vi "HDF5_Init_Tone_Refs_20171218_1427.vi"(5 "HDF5 file ref":T2 format="%.0x", 9 "File Exists?":bool, 11 "error in":errorcluster) -> (3 "ComplexRefs":T1[](array[typedef]) {"Group_ref" format="%.0x"; "QSpect_dset" format="%.0x"; "ISpect_dset" format="%.0x"; "PwrSpect_dset" format="%.0x"; "TImeStamp_dset" format="%.0x"}, 4 "ToneRefs":T3[](array[typedef]) {"Group_ref" format="%.0x"; "Cal"."Downshift_dset" format="%.0x"; "Cal"."DeltaPhase_dset" format="%.0x"; "Cal"."Phase_dset" format="%.0x"; "Cal"."SNR_dset" format="%.0x"; "Cal"."df_dset" format="%.0x"; "Cal"."PeakLoc_dset" format="%.0x"; "Cal"."MaxValue_dset" format="%.0x"; "Cal"."TImeStamp_dset" format="%.0x"; "Cal"."TimeString_dset" format="%.0x"; "Beac"."Downshift_dset" format="%.0x"; "Beac"."DeltaPhase_dset" format="%.0x"; "Beac"."Phase_dset" format="%.0x"; "Beac"."SNR_dset" format="%.0x"; "Beac"."df_dset" format="%.0x"; "Beac"."PeakLoc_dset" format="%.0x"; "Beac"."MaxValue_dset" format="%.0x"; "Beac"."TImeStamp_dset" format="%.0x"; "Beac"."TimeString_dset" format="%.0x"; "CalZoom_dSet" format="%.0x"; "BeacZoom_dSet" format="%.0x"}, 6 "HDF5 file ref":T2 format="%.0x", 15 "error out":errorcluster)   [LabVIEW 2018]
doc: "Set up the HDF5 data structure and initialize the references for the Tone1, Tone2, Tone3, and Tone4 Groups and the datasets (tables) within each Group.\n\nData structure:\nTone1 (Group) \n Beac - cluster (Dataset)\n BeacZoom - 1024 element Double array (waveform) \n Cal - cluster\n CalZoom - 1024 element Double array (waveform) \nTone2\n Beac - cluster\n BeacZoom - 1024 element Double array (waveform) \n Cal - cluster\n CalZoom - 1024 element Double array (waveform) \nTone3\n Beac - cluster\n BeacZoom - 1024 element Double array (waveform) \n Cal - cluster\n CalZoom - 1024 element Double array (waveform) \nTone4\n Beac - cluster\n BeacZoom - 1024 element Double array (waveform) \n Cal - cluster\n CalZoom - 1024 element Double array (waveform)"
uses:
  Controls/Clusts/ToneGroupRefsClust.ctl
  <vilib>/addons/h5labview2/base/hid_t.ctl
  HDF5_Tone_refs.ctl
  HDF5_Complex_Refs.ctl
  lib_path_mod_20200519.vi
  <vilib>/addons/h5labview2/base/H5Equery.vi
  <vilib>/addons/h5labview2/attrib/H5Awrite.llb/H5Awrite.xnode
  <vilib>/addons/h5labview2/group/H5G.lvlib
  <vilib>/addons/h5labview2/dataset/H5D.lvlib
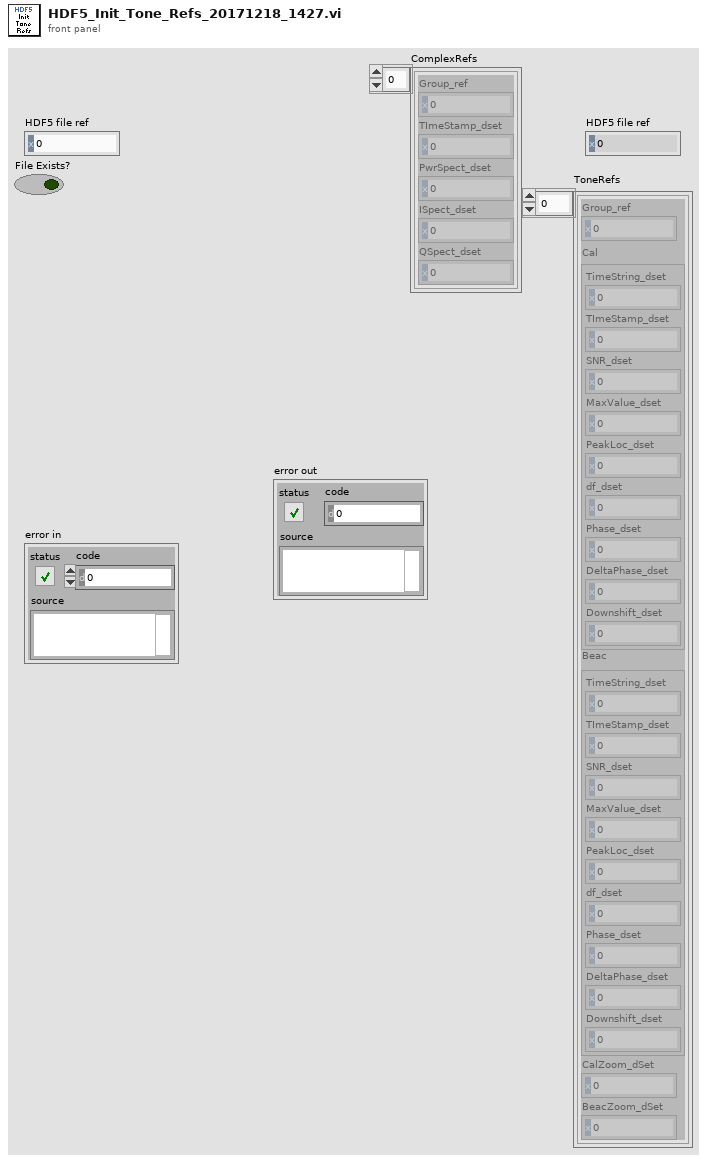
[diagram p1: front panel]
types:
  T1 = typedef "HDF5_Complex_Refs.ctl" = cluster{"Group_ref":T2, "TImeStamp_dset":T2, "PwrSpect_dset":T2, "ISpect_dset":T2, "QSpect_dset":T2}
  T2 = typedef "hid_t.ctl" = i32
  T3 = typedef "ToneGroupRefsClust.ctl" = cluster{"Group_ref":T2, "Cal":T4, "Beac":T4, "CalZoom_dSet":T2, "BeacZoom_dSet":T2}
  T4 = typedef "HDF5_Tone_refs.ctl" = cluster{"TimeString_dset":T2, "TImeStamp_dset":T2, "SNR_dset":T2, "MaxValue_dset":T2, "PeakLoc_dset":T2, "df_dset":T2, "Phase_dset":T2, "DeltaPhase_dset":T2, "Downshift_dset":T2}
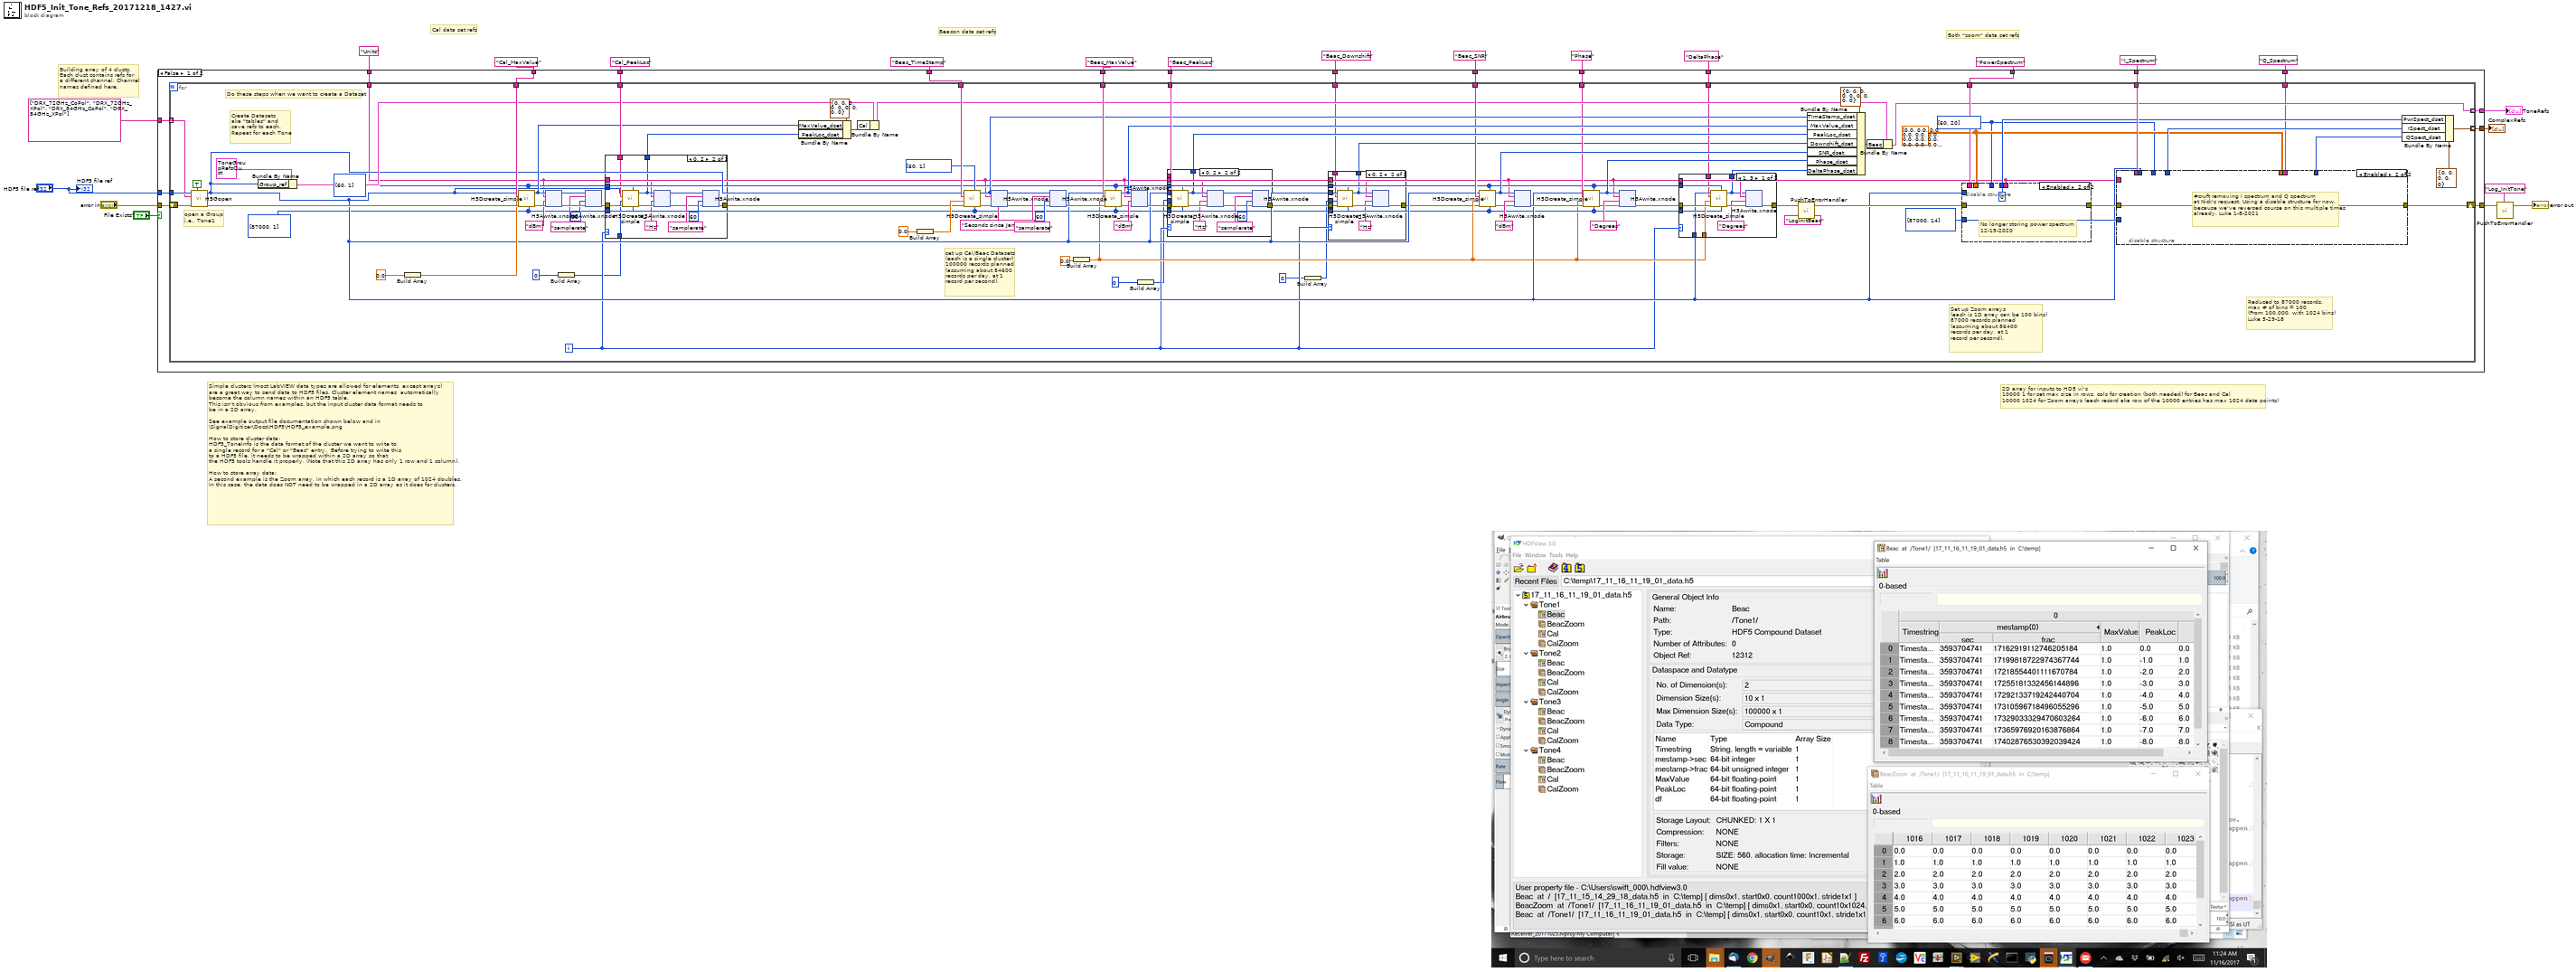
[diagram p0: block diagram]
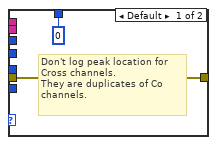
[diagram p2: hidden frame]
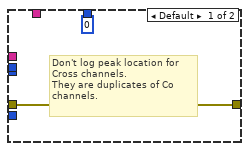
[diagram p3: hidden frame]
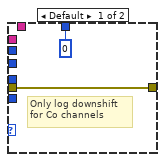
[diagram p4: hidden frame]
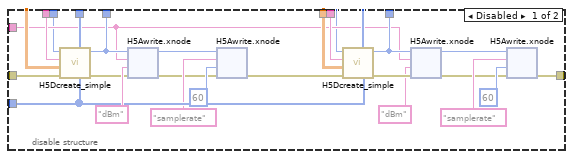
[diagram p5: hidden frame]
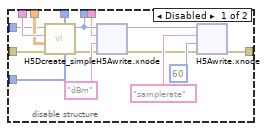
[diagram p6: hidden frame]
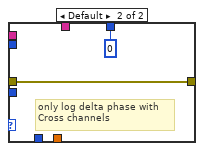
[diagram p7: hidden frame]
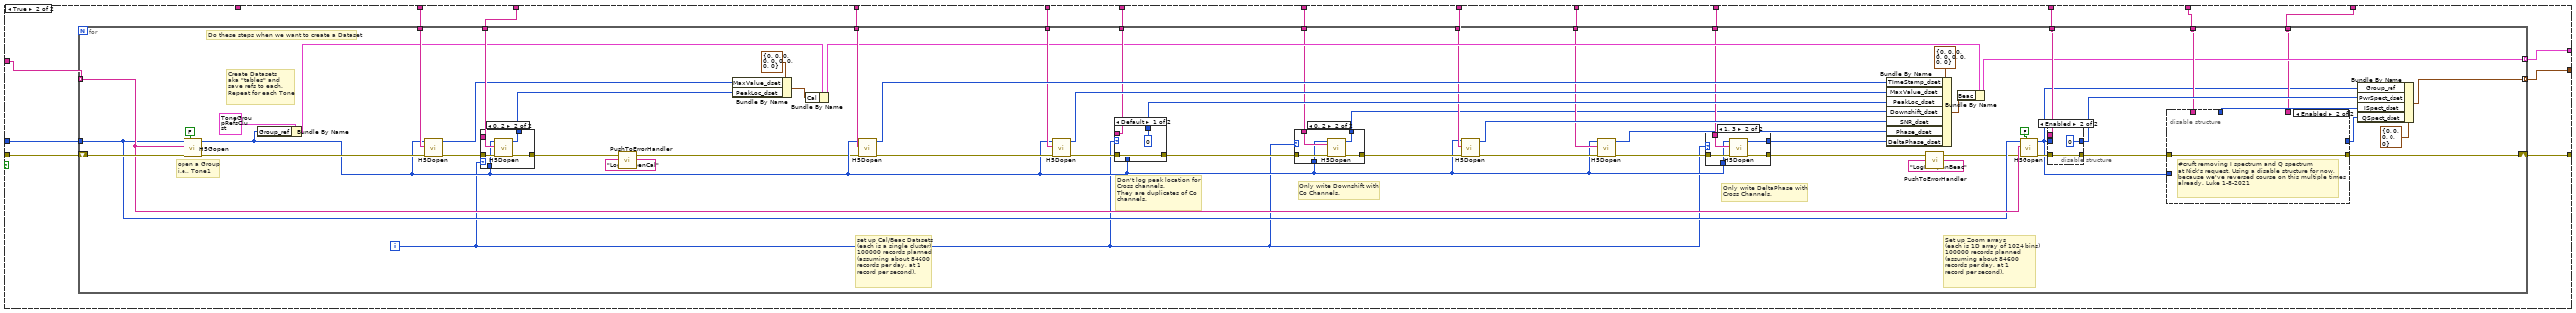
[diagram p8: hidden frame]
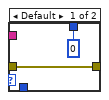
[diagram p9: hidden frame]
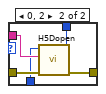
[diagram p10: hidden frame]
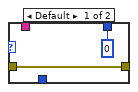
[diagram p11: hidden frame]
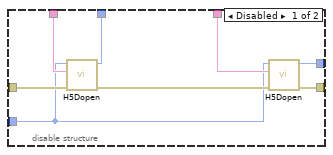
[diagram p12: hidden frame]
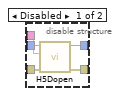
[diagram p13: hidden frame]
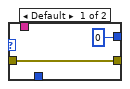
[diagram p14: hidden frame]
diagram:
  # "Both \"zoom\" data set refs"
  # "Beacon data set refs"
  # "Cal data set refs"
  # "Building array of 4 clusts.\nEach clust contains refs for \na different channel. Channel\nnames defined here."
  # "Simple clusters (most LabVIEW data types are allowed for elements, except arrays) \nare a great way to send data to HDF5 files. Cluster element names  automatically\nbecome the column names within an HDF5 table.\nThis isn't obvious from examples, but the input cluster data format needs to \nbe in a 2D array.\n\nSee example output file documentation shown below and in\n\\SignalDigitizer\\Docs\\HDF5\\HDF5_example.png\n\nHow to store cluster data:\nHDF5_ToneInfo is the data format of the cluster we want to write to \na single record for a \"Cal\" or \"Beac\" entry.  Before trying to write this \nto a HDF5 file, it needs to be wrapped within a 2D array so that \nthe HDF5 tools handle it properly. (Note that this 2D array has only 1 row and 1 column).\n\nHow to store array data:\nA second example is the Zoom array, in which each record is a 1D array of 1024 doubles.\nIn this case, the data does NOT need to be wrapped in a 2D array as it does for clusters."
  # "2D array for inputs to HD5 vi's\n10000 1 for set max size in rows, cols for creation (both needed) for Beac and Cal\n10000 1024 for Zoom arrays (each record aka row of the 10000 entries has max 1024 data points)"
  n1 = case shown="False" "File Exists?" {
    tunnel: [w41 w613] -> w22
    tunnel: "error in" -> [w40 w612]
    tunnel: "HDF5 file ref" -> [w39 w611]
    tunnel: string[] ["DRX_72GHz_CoPol", "DRX_72GHz_XPol", "DRX_84GHz_CoPol", "DRX_84GHz_XPol"] -> [w38 w610]
    tunnel: [w37 w609] -> w7
    tunnel: "PowerSpectrum" ("string") -> [w36 w608]
    tunnel: "I_Spectrum" ("string") -> [w35 w607]
    tunnel: "Cal_MaxValue" ("string") -> [w34 w606]
    tunnel: "Cal_PeakLoc" ("string") -> [w33 w605]
    tunnel: "Beac_TimeStamp" ("string") -> [w32 w604]
    tunnel: "Beac_MaxValue" ("string") -> [w31 w603]
    tunnel: "Beac_PeakLoc" ("string") -> [w30 w602]
    tunnel: "Units" ("attrib name") -> [w29 _]
    tunnel: [w28 w601] -> w9
    tunnel: "Q_Spectrum" ("string") -> [w27 w600]
    tunnel: "Beac_SNR" ("string") -> [w26 w599]
    tunnel: "Phase" ("string") -> [w25 w598]
    tunnel: "DeltaPhase" ("string") -> [w24 w597]
    tunnel: "Beac_Downshift" ("string") -> [w23 w596]
    frame False {
      n2 = for {
        tunnel: w39 -> [w132]
        shift-right: [w77] -> w37
        shift-left: w40 -> [w130]
        tunnel: w38 -> [w129] mode=indexing
        tunnel: [w96] -> w41 mode=indexing
        tunnel: w36 -> [w128]
        tunnel: w35 -> [w127]
        tunnel: w34 -> [w126]
        tunnel: w33 -> [w125]
        tunnel: w32 -> [w124]
        tunnel: w31 -> [w123]
        tunnel: w30 -> [w122]
        tunnel: w29 -> [w52]
        tunnel: [w94] -> w28 mode=indexing
        tunnel: w27 -> [w89]
        tunnel: w26 -> [w72]
        tunnel: w25 -> [w61]
        tunnel: w24 -> [w60]
        tunnel: w23 -> [w56]
        i -> [w48]
        w90 = u64[] [87000, 14] ("ZoomArraySize")
        w92 = u64[] [60, 20] ("chunk size")
        w53 = u64[] [60, 1] ("chunk size")
        w54 = u64[] [87000, 1] ("CalBeacArraySize")
        w93 = sgl[][] [[0.0, 0.0, 0.0, 0.0, 0.0, 0.0, 0.0, 0.0, 0.0, 0.0, 0.0, 0.0, 0.0, 0.0, 0.0, 0.0, 0.0, 0.0, 0.0, 0.0, 0.0, 0.0, 0.0, 0.0, 0.0, 0.0, 0.0, 0.0, 0.0, 0.0, 0.0, 0.0, 0.0, 0.0, 0.0, 0.0, 0.0, 0.0, 0.0, 0.0, 0.0, 0.0, 0.0, 0.0, 0.0, 0.0, 0.0, 0.0, 0.0, 0.0, 0.0, 0.0, 0.0, 0.0, 0.0, 0.0, 0.0, 0.0, 0.0, 0.0, 0.0, 0.0, 0.0, 0.0, 0.0, 0.0, 0.0, 0.0, 0.0, 0.0, 0.0, 0.0, 0.0, 0.0, 0.0, 0.0, 0.0, 0.0, 0.0, 0.0, 0.0, 0.0, 0.0, 0.0, 0.0, 0.0, 0.0, 0.0, 0.0, 0.0, 0.0, 0.0, 0.0, 0.0, 0.0, 0.0, 0.0, 0.0, 0.0, 0.0, 0.0, 0.0, 0.0, 0.0, 0.0, 0.0, 0.0, 0.0, 0.0, 0.0, 0.0, 0.0, 0.0, 0.0, 0.0, 0.0, 0.0, 0.0, 0.0, 0.0, 0.0, 0.0, 0.0, 0.0, 0.0, 0.0, 0.0, 0.0, 0.0, 0.0, 0.0, 0.0, 0.0, 0.0, 0.0, 0.0, 0.0, 0.0, 0.0, 0.0, 0.0, 0.0, 0.0, 0.0, 0.0, 0.0, 0.0, 0.0, 0.0, 0.0, 0.0, 0.0, 0.0, 0.0, 0.0, 0.0, 0.0, 0.0, 0.0, 0.0, 0.0, 0.0, 0.0, 0.0, 0.0, 0.0, 0.0, 0.0, 0.0, 0.0, 0.0, 0.0, 0.0, 0.0, 0.0, 0.0, 0.0, 0.0, 0.0, 0.0, 0.0, 0.0, 0.0, 0.0, 0.0, 0.0, 0.0, 0.0, 0.0, 0.0, 0.0, 0.0, 0.0, 0.0, 0.0, 0.0, 0.0, 0.0, 0.0, 0.0, 0.0, 0.0, 0.0, 0.0, 0.0, 0.0, 0.0, 0.0, 0.0, 0.0, 0.0, 0.0, 0.0, 0.0, 0.0, 0.0, 0.0, 0.0, 0.0, 0.0, 0.0, 0.0, 0.0, 0.0, 0.0, 0.0, 0.0, 0.0, 0.0, 0.0, 0.0, 0.0, 0.0, 0.0, 0.0, 0.0, 0.0, 0.0, 0.0, 0.0, 0.0, 0.0, 0.0, 0.0, 0.0, 0.0, 0.0, 0.0, 0.0, 0.0, 0.0, 0.0, 0.0, 0.0, 0.0, 0.0, 0.0, 0.0, 0.0, 0.0, 0.0, 0.0, 0.0, 0.0, 0.0, 0.0, 0.0, 0.0, 0.0, 0.0, 0.0, 0.0, 0.0, 0.0, 0.0, 0.0, 0.0, 0.0, 0.0, 0.0, 0.0, 0.0, 0.0, 0.0, 0.0, 0.0, 0.0, 0.0, 0.0, 0.0, 0.0, 0.0, 0.0, 0.0, 0.0, 0.0, 0.0, 0.0, 0.0, 0.0, 0.0, 0.0, 0.0, 0.0, 0.0, 0.0, 0.0, 0.0, 0.0, 0.0, 0.0, 0.0, 0.0, 0.0, 0.0, 0.0, 0.0, 0.0, 0.0, 0.0, 0.0, 0.0, 0.0, 0.0, 0.0, 0.0, 0.0, 0.0, 0.0, 0.0, 0.0, 0.0, 0.0, 0.0, 0.0, 0.0, 0.0, 0.0, 0.0, 0.0, 0.0, 0.0, 0.0, 0.0, 0.0, 0.0, 0.0, 0.0, 0.0, 0.0, 0.0, 0.0, 0.0, 0.0, 0.0, 0.0, 0.0, 0.0, 0.0, 0.0, 0.0, 0.0, 0.0, 0.0, 0.0, 0.0, 0.0, 0.0, 0.0, 0.0, 0.0, 0.0, 0.0, 0.0, 0.0, 0.0, 0.0, 0.0, 0.0, 0.0, 0.0, 0.0, 0.0, 0.0, 0.0, 0.0, 0.0, 0.0, 0.0, 0.0, 0.0, 0.0, 0.0, 0.0, 0.0, 0.0, 0.0, 0.0, 0.0, 0.0, 0.0, 0.0, 0.0, 0.0, 0.0, 0.0, 0.0, 0.0, 0.0, 0.0, 0.0, 0.0, 0.0, 0.0, 0.0, 0.0, 0.0, 0.0, 0.0, 0.0, 0.0, 0.0, 0.0, 0.0, 0.0, 0.0, 0.0, 0.0, 0.0, 0.0, 0.0, 0.0, 0.0, 0.0, 0.0, 0.0, 0.0, 0.0, 0.0, 0.0, 0.0, 0.0, 0.0, 0.0, 0.0, 0.0, 0.0, 0.0, 0.0, 0.0, 0.0, 0.0, 0.0, 0.0, 0.0, 0.0, 0.0, 0.0, 0.0, 0.0, 0.0, 0.0, 0.0, 0.0, 0.0, 0.0, 0.0, 0.0, 0.0, 0.0, 0.0, 0.0, 0.0, 0.0, 0.0, 0.0, 0.0, 0.0, 0.0, 0.0, 0.0, 0.0, 0.0, 0.0, 0.0, 0.0, 0.0, 0.0, 0.0, 0.0, 0.0, 0.0, 0.0, 0.0, 0.0, 0.0, 0.0, 0.0, 0.0, 0.0, 0.0, 0.0, 0.0, 0.0, 0.0, 0.0, 0.0, 0.0, 0.0, 0.0, 0.0, 0.0, 0.0, 0.0, 0.0, 0.0, 0.0, 0.0, 0.0, 0.0, 0.0, 0.0, 0.0, 0.0, 0.0, 0.0, 0.0, 0.0, 0.0, 0.0, 0.0, 0.0, 0.0, 0.0, 0.0, 0.0, 0.0, 0.0, 0.0, 0.0, 0.0, 0.0, 0.0, 0.0, 0.0, 0.0, 0.0, 0.0, 0.0, 0.0, 0.0, 0.0, 0.0, 0.0, 0.0, 0.0, 0.0, 0.0, 0.0, 0.0, 0.0, 0.0, 0.0, 0.0, 0.0, 0.0, 0.0, 0.0, 0.0, 0.0, 0.0, 0.0, 0.0, 0.0, 0.0, 0.0, 0.0, 0.0, 0.0, 0.0, 0.0, 0.0, 0.0, 0.0, 0.0, 0.0, 0.0, 0.0, 0.0, 0.0, 0.0, 0.0, 0.0, 0.0, 0.0, 0.0, 0.0, 0.0, 0.0, 0.0, 0.0, 0.0, 0.0, 0.0, 0.0, 0.0, 0.0, 0.0, 0.0, 0.0, 0.0, 0.0, 0.0, 0.0, 0.0, 0.0, 0.0, 0.0, 0.0, 0.0, 0.0, 0.0, 0.0, 0.0, 0.0, 0.0, 0.0, 0.0, 0.0, 0.0, 0.0, 0.0, 0.0, 0.0, 0.0, 0.0, 0.0, 0.0, 0.0, 0.0, 0.0, 0.0, 0.0, 0.0, 0.0, 0.0, 0.0, 0.0, 0.0, 0.0, 0.0, 0.0, 0.0, 0.0, 0.0, 0.0, 0.0, 0.0, 0.0, 0.0, 0.0, 0.0, 0.0, 0.0, 0.0, 0.0, 0.0, 0.0, 0.0, 0.0, 0.0, 0.0, 0.0, 0.0, 0.0, 0.0, 0.0, 0.0, 0.0, 0.0, 0.0, 0.0, 0.0, 0.0, 0.0, 0.0, 0.0, 0.0, 0.0, 0.0, 0.0, 0.0, 0.0, 0.0, 0.0, 0.0, 0.0, 0.0, 0.0, 0.0, 0.0, 0.0, 0.0, 0.0, 0.0, 0.0, 0.0, 0.0, 0.0, 0.0, 0.0, 0.0, 0.0, 0.0, 0.0, 0.0, 0.0, 0.0, 0.0, 0.0, 0.0, 0.0, 0.0, 0.0, 0.0, 0.0, 0.0, 0.0, 0.0, 0.0, 0.0, 0.0, 0.0, 0.0, 0.0, 0.0, 0.0, 0.0, 0.0, 0.0, 0.0, 0.0, 0.0, 0.0, 0.0, 0.0, 0.0, 0.0, 0.0, 0.0, 0.0, 0.0, 0.0, 0.0, 0.0, 0.0, 0.0, 0.0, 0.0, 0.0, 0.0, 0.0, 0.0, 0.0, 0.0, 0.0, 0.0, 0.0, 0.0, 0.0, 0.0, 0.0, 0.0, 0.0, 0.0, 0.0, 0.0, 0.0, 0.0, 0.0, 0.0, 0.0, 0.0, 0.0, 0.0, 0.0, 0.0, 0.0, 0.0, 0.0, 0.0, 0.0, 0.0, 0.0, 0.0, 0.0, 0.0, 0.0, 0.0, 0.0, 0.0, 0.0, 0.0, 0.0, 0.0, 0.0, 0.0, 0.0, 0.0, 0.0, 0.0, 0.0, 0.0, 0.0, 0.0, 0.0, 0.0, 0.0, 0.0, 0.0, 0.0, 0.0, 0.0, 0.0, 0.0, 0.0, 0.0, 0.0, 0.0, 0.0, 0.0, 0.0, 0.0, 0.0, 0.0, 0.0, 0.0, 0.0, 0.0, 0.0, 0.0, 0.0, 0.0, 0.0, 0.0, 0.0, 0.0, 0.0, 0.0, 0.0, 0.0, 0.0, 0.0, 0.0, 0.0, 0.0, 0.0, 0.0, 0.0, 0.0, 0.0, 0.0, 0.0, 0.0, 0.0, 0.0, 0.0, 0.0, 0.0, 0.0, 0.0, 0.0, 0.0, 0.0, 0.0, 0.0, 0.0, 0.0, 0.0, 0.0, 0.0, 0.0, 0.0, 0.0, 0.0, 0.0, 0.0, 0.0, 0.0, 0.0, 0.0, 0.0, 0.0, 0.0, 0.0, 0.0, 0.0, 0.0, 0.0, 0.0, 0.0, 0.0, 0.0, 0.0, 0.0, 0.0, 0.0, 0.0, 0.0, 0.0, 0.0, 0.0, 0.0, 0.0, 0.0, 0.0, 0.0, 0.0, 0.0, 0.0, 0.0, 0.0, 0.0, 0.0, 0.0, 0.0, 0.0, 0.0, 0.0, 0.0, 0.0, 0.0, 0.0, 0.0, 0.0, 0.0, 0.0, 0.0, 0.0, 0.0, 0.0, 0.0, 0.0, 0.0, 0.0, 0.0, 0.0, 0.0, 0.0, 0.0, 0.0, 0.0, 0.0, 0.0, 0.0, 0.0, 0.0, 0.0, 0.0, 0.0, 0.0, 0.0, 0.0, 0.0, 0.0, 0.0, 0.0, 0.0, 0.0, 0.0, 0.0, 0.0, 0.0, 0.0, 0.0, 0.0, 0.0, 0.0, 0.0, 0.0, 0.0, 0.0, 0.0, 0.0, 0.0, 0.0, 0.0, 0.0, 0.0, 0.0, 0.0, 0.0, 0.0, 0.0, 0.0, 0.0, 0.0, 0.0, 0.0, 0.0, 0.0, 0.0, 0.0, 0.0, 0.0, 0.0, 0.0, 0.0, 0.0, 0.0, 0.0, 0.0, 0.0, 0.0, 0.0, 0.0, 0.0, 0.0, 0.0, 0.0, 0.0, 0.0, 0.0, 0.0]] ("Zoom")
        # "Reduced to 87000 records,\nmax # of bins = 100\n(From 100,000, with 1024 bins)\nLuke 5-29-18"
        # "Do these steps when we want to create a Dataset"
        # "Create Datasets\naka \"tables\" and\nsave refs to each.\nRepeat for each Tone"
        # "Set up Zoom arrays\n(each is 1D array can be 100 bins)\n87000 records planned\n(assuming about 86400\nrecords per day, at 1\nrecord per second)."
        # "set up Cal/Beac Datasets\n(each is a single cluster)\n100000 records planned\n(assuming about 84600\nrecords per day, at 1\nrecord per second)."
        # "open a Group\ni.e., Tone1"
        n3 = call <vilib>:"H5Gopen.vi"("create? (F)"=TRUE, "error in (no error)"=w130, "name"=w129, "ref in"=w132) -> ("error out"=w115:errorcluster, "group out"=w57:T2)  [unwired: 6 in]
        n4 = Bundle By Name(cluster=T3 {"Group_ref"=0, "Cal"={"TimeString_dset"=0, "TImeStamp_dset"=0, "SNR_dset"=0, "MaxValue_dset"=0, "PeakLoc_dset"=0, "df_dset"=0, "Phase_dset"=0, "DeltaPhase_dset"=0, "Downshift_dset"=0}, "Beac"={"TimeString_dset"=0, "TImeStamp_dset"=0, "SNR_dset"=0, "MaxValue_dset"=0, "PeakLoc_dset"=0, "df_dset"=0, "Phase_dset"=0, "DeltaPhase_dset"=0, "Downshift_dset"=0}, "CalZoom_dSet"=0, "BeacZoom_dSet"=0}, "Group_ref"=w57) -> (w119:T3)
        n5 = Build Array(sgl 0.0) -> (w70:sgl[])
        n6 = call <vilib>:"H5Dcreate_simple.vi"("max size"=w54, "chunk size"=w53, "error in (no error)"=w115, "type in"=w70, "name"=w126, "ref in"=w57) -> ("error out"=w114:errorcluster, "dset out"=w76:T2)  [unwired: 4 in]
        n7 = xnode "H5Awrite.xnode"("error in (no error)"=w114, "data"="dBm", "attrib name"=w52, "ref in"=w76) -> ("error out"=w88:errorcluster, "ref out"=w86:i32)  [unwired: 3 in, 1 out]
        n8 = Build Array(0) -> (w46:i32[])
        n9 = xnode "H5Awrite.xnode"("error in (no error)"=w88, "data"=u32 60, "attrib name"="samplerate", "ref in"=w86) -> ("error out"=w87:errorcluster)  [unwired: 3 in, 2 out]
        n10 = case shown="0, 2" w48 {
          tunnel: w125 -> [_ w204]
          tunnel: [T2 0 ("dset out") w201] -> w108
          tunnel: w87 -> [w189 w200]
          tunnel: w46 -> [_ w196]
          tunnel: [w189 w194] -> w67
          tunnel: w57 -> [_ w193]
          tunnel: w54 -> [_ w192]
          tunnel: w53 -> [_ w191]
          tunnel: w52 -> [_ w190]
          frame Default {
            # "Don't log peak location for \nCross channels. \nThey are duplicates of Co\nchannels."
          }
          frame 0, 2 {
            n11 = call <vilib>:"H5Dcreate_simple.vi"("max size"=w192, "chunk size"=w191, "error in (no error)"=w200, "type in"=w196, "name"=w204, "ref in"=w193) -> ("error out"=w203:errorcluster, "dset out"=w201:T2)  [unwired: 4 in]
            n12 = xnode "H5Awrite.xnode"("error in (no error)"=w203, "data"="Hz", "attrib name"=w190, "ref in"=w201) -> ("error out"=w195:errorcluster, "ref out"=w197:i32)  [unwired: 3 in, 1 out]
            n13 = xnode "H5Awrite.xnode"("error in (no error)"=w195, "data"=u32 60, "attrib name"="samplerate", "ref in"=w197) -> ("error out"=w194:errorcluster)  [unwired: 3 in, 2 out]
          }
        }
        n14 = Bundle By Name(cluster=T4 {"TimeString_dset"=0, "TImeStamp_dset"=0, "SNR_dset"=0, "MaxValue_dset"=0, "PeakLoc_dset"=0, "df_dset"=0, "Phase_dset"=0, "DeltaPhase_dset"=0, "Downshift_dset"=0} ("Cal"), "MaxValue_dset"=w76, "PeakLoc_dset"=w108) -> (w118:T4)
        n15 = Bundle By Name(cluster=w119, "Cal"=w118) -> (w71:T3)
        n16 = Build Array(0.0 ("Timestamp")) -> (w98:dbl[])
        n17 = call <vilib>:"H5Dcreate_simple.vi"("max size"=w54, "chunk size"=u64[] [60, 1], "error in (no error)"=w67, "type in"=w98, "name"=w124, "ref in"=w57) -> ("error out"=w113:errorcluster, "dset out"=w107:T2)  [unwired: 4 in]
        n18 = xnode "H5Awrite.xnode"("error in (no error)"=w113, "data"="Seconds since Jan 1, 1904", "attrib name"=w52, "ref in"=w107) -> ("error out"=w81:errorcluster, "ref out"=w80:i32)  [unwired: 3 in, 1 out]
        n19 = xnode "H5Awrite.xnode"("error in (no error)"=w81, "data"=u32 60, "attrib name"="samplerate", "ref in"=w80) -> ("error out"=w79:errorcluster)  [unwired: 3 in, 2 out]
        n20 = Build Array(sgl 0.0) -> (w51:sgl[])
        n21 = call <vilib>:"H5Dcreate_simple.vi"("max size"=w54, "chunk size"=w53, "error in (no error)"=w79, "type in"=w51, "name"=w123, "ref in"=w57) -> ("error out"=w102:errorcluster, "dset out"=w106:T2)  [unwired: 4 in]
        n22 = xnode "H5Awrite.xnode"("error in (no error)"=w102, "data"="dBm", "attrib name"=w52, "ref in"=w106) -> ("error out"=w112:errorcluster)  [unwired: 3 in, 2 out]
        n23 = Build Array(0) -> (w44:i32[])
        n24 = case shown="0, 2" w48 {
          tunnel: w122 -> [_ w149]
          tunnel: w112 -> [w134 w148]
          tunnel: [T2 0 ("dset out") w145] -> w105
          tunnel: w57 -> [_ w140]
          tunnel: w54 -> [_ w139]
          tunnel: w53 -> [_ w138]
          tunnel: w52 -> [_ w137]
          tunnel: w44 -> [_ w136]
          tunnel: [w134 w135] -> w50
          frame Default {
            # "Don't log peak location for \nCross channels. \nThey are duplicates of Co\nchannels."
          }
          frame 0, 2 {
            n25 = call <vilib>:"H5Dcreate_simple.vi"("max size"=w139, "chunk size"=w138, "error in (no error)"=w148, "type in"=w136, "name"=w149, "ref in"=w140) -> ("error out"=w147:errorcluster, "dset out"=w145:T2)  [unwired: 4 in]
            n26 = xnode "H5Awrite.xnode"("error in (no error)"=w147, "data"="Hz", "attrib name"=w137, "ref in"=w145) -> ("error out"=w142:errorcluster, "ref out"=w141:i32)  [unwired: 3 in, 1 out]
            n27 = xnode "H5Awrite.xnode"("error in (no error)"=w142, "data"=u32 60, "attrib name"="samplerate", "ref in"=w141) -> ("error out"=w135:errorcluster)  [unwired: 3 in, 2 out]
          }
        }
        n28 = Build Array(0) -> (w42:i32[])
        n29 = case shown="0, 2" w48 {
          tunnel: w57 -> [_ w291]
          tunnel: w56 -> [_ w290]
          tunnel: [T2 0 ("dset out") w289] -> w55
          tunnel: w54 -> [_ w288]
          tunnel: w53 -> [_ w287]
          tunnel: w52 -> [_ w286]
          tunnel: w42 -> [_ w285]
          tunnel: w50 -> [w281 w284]
          tunnel: [w281 w283] -> w49
          frame Default {
            # "Only log downshift\nfor Co channels"
          }
          frame 0, 2 {
            n30 = call <vilib>:"H5Dcreate_simple.vi"("max size"=w288, "chunk size"=w287, "error in (no error)"=w284, "type in"=w285, "name"=w290, "ref in"=w291) -> ("error out"=w293:errorcluster, "dset out"=w289:T2)  [unwired: 4 in]
            n31 = xnode "H5Awrite.xnode"("error in (no error)"=w293, "data"="Hz", "attrib name"=w286, "ref in"=w289) -> ("error out"=w283:errorcluster)  [unwired: 3 in, 2 out]
          }
        }
        n32 = call <vilib>:"H5Dcreate_simple.vi"("max size"=w54, "chunk size"=w53, "error in (no error)"=w49, "type in"=w51, "name"=w72, "ref in"=w57) -> ("error out"=w74:errorcluster, "dset out"=w73:T2)  [unwired: 4 in]
        n33 = xnode "H5Awrite.xnode"("error in (no error)"=w74, "data"="dBm", "attrib name"=w52, "ref in"=w73) -> ("error out"=w59:errorcluster)  [unwired: 3 in, 2 out]
        n34 = call <vilib>:"H5Dcreate_simple.vi"("max size"=w54, "chunk size"=w53, "error in (no error)"=w59, "type in"=w51, "name"=w61, "ref in"=w57) -> ("error out"=w64:errorcluster, "dset out"=w63:T2)  [unwired: 4 in]
        n35 = xnode "H5Awrite.xnode"("error in (no error)"=w64, "data"="Degrees", "attrib name"=w52, "ref in"=w63) -> ("error out"=w66:errorcluster)  [unwired: 3 in, 2 out]
        n36 = case shown="1, 3" w48 {
          tunnel: w66 -> [w477 w499]
          tunnel: w52 -> [w476 _]
          tunnel: [w475 T2 0 ("dset out")] -> w62
          tunnel: w53 -> [w474 _]
          tunnel: w51 -> [w473 _]
          tunnel: w54 -> [w472 _]
          tunnel: w57 -> [w471 _]
          tunnel: w60 -> [w470 _]
          tunnel: [w469 w499] -> w58
          frame 1, 3 {
            n37 = call <vilib>:"H5Dcreate_simple.vi"("max size"=w472, "chunk size"=w474, "error in (no error)"=w477, "type in"=w473, "name"=w470, "ref in"=w471) -> ("error out"=w479:errorcluster, "dset out"=w475:T2)  [unwired: 4 in]
            n38 = xnode "H5Awrite.xnode"("error in (no error)"=w479, "data"="Degrees", "attrib name"=w476, "ref in"=w475) -> ("error out"=w469:errorcluster)  [unwired: 3 in, 2 out]
          }
          frame Default {
            # "only log delta phase with \nCross channels"
          }
        }
        n39 = call "PushToErrorHandler.vi"("ErrorIn"=w58, "ErrorLocation"="LogInitBeac") -> ("ErrorOut"=w69:errorcluster)  [unwired: 5 in]
        n40 = Bundle By Name(cluster=T4 {"TimeString_dset"=0, "TImeStamp_dset"=0, "SNR_dset"=0, "MaxValue_dset"=0, "PeakLoc_dset"=0, "df_dset"=0, "Phase_dset"=0, "DeltaPhase_dset"=0, "Downshift_dset"=0} ("Cal"), "TImeStamp_dset"=w107, "MaxValue_dset"=w106, "PeakLoc_dset"=w105, "Downshift_dset"=w55, "SNR_dset"=w73, "Phase_dset"=w63, "DeltaPhase_dset"=w62) -> (w117:T4)
        n41 = Bundle By Name(cluster=w71, "Beac"=w117) -> (w96:T3)
        n42 = disable-structure shown="Enabled" {
          disable-tunnel: w128 -> [w428 _]
          disable-tunnel: [w427 T2 0 ("dset out")] -> w104
          disable-tunnel: w93 -> [w424 _]
          disable-tunnel: w92 -> [w423 _]
          disable-tunnel: w90 -> [w422 _]
          disable-tunnel: [w417 w468] -> w78
          disable-tunnel: w69 -> [w416 w468]
          disable-tunnel: w52 -> [w415 _]
          disable-tunnel: w57 -> [w414 _]
          frame Disabled {
            n43 = call <vilib>:"H5Dcreate_simple.vi"("max size"=w422, "chunk size"=w423, "error in (no error)"=w416, "type in"=w424, "name"=w428, "ref in"=w414) -> ("error out"=w425:errorcluster, "dset out"=w427:T2)  [unwired: 4 in]
            n44 = xnode "H5Awrite.xnode"("error in (no error)"=w425, "data"="dBm", "attrib name"=w415, "ref in"=w427) -> ("error out"=w419:errorcluster, "ref out"=w418:i32)  [unwired: 3 in, 1 out]
            n45 = xnode "H5Awrite.xnode"("error in (no error)"=w419, "data"=u32 60, "attrib name"="samplerate", "ref in"=w418) -> ("error out"=w417:errorcluster)  [unwired: 3 in, 2 out]
          }
          frame Enabled {
            # "No longer storing power spectrum\n12-15-2020"
          }
        }
        n46 = disable-structure shown="Enabled" {
          disable-tunnel: w127 -> [w336 _]
          disable-tunnel: [w335 _] -> w103
          disable-tunnel: w93 -> [w330 _]
          disable-tunnel: w92 -> [w329 _]
          disable-tunnel: [w328 _] -> w91
          disable-tunnel: w90 -> [w327 _]
          disable-tunnel: w89 -> [w326 _]
          disable-tunnel: w78 -> [w325 w413]
          disable-tunnel: [w315 w413] -> w77
          disable-tunnel: w52 -> [w314 _]
          disable-tunnel: w57 -> [w313 _]
          frame Disabled {
            n47 = call <vilib>:"H5Dcreate_simple.vi"("max size"=w327, "chunk size"=w329, "error in (no error)"=w325, "type in"=w330, "name"=w336, "ref in"=w313) -> ("error out"=w333:errorcluster, "dset out"=w335:T2)  [unwired: 4 in]
            n48 = xnode "H5Awrite.xnode"("error in (no error)"=w333, "data"="dBm", "attrib name"=w314, "ref in"=w335) -> ("error out"=w322:errorcluster, "ref out"=w321:i32)  [unwired: 3 in, 1 out]
            n49 = xnode "H5Awrite.xnode"("error in (no error)"=w322, "data"=u32 60, "attrib name"="samplerate", "ref in"=w321) -> ("error out"=w320:errorcluster)  [unwired: 3 in, 2 out]
            n50 = call <vilib>:"H5Dcreate_simple.vi"("max size"=w327, "chunk size"=w329, "error in (no error)"=w320, "type in"=w330, "name"=w326, "ref in"=w313) -> ("error out"=w332:errorcluster, "dset out"=w328:T2)  [unwired: 4 in]
            n51 = xnode "H5Awrite.xnode"("error in (no error)"=w332, "data"="dBm", "attrib name"=w314, "ref in"=w328) -> ("error out"=w317:errorcluster, "ref out"=w316:i32)  [unwired: 3 in, 1 out]
            n52 = xnode "H5Awrite.xnode"("error in (no error)"=w317, "data"=u32 60, "attrib name"="samplerate", "ref in"=w316) -> ("error out"=w315:errorcluster)  [unwired: 3 in, 2 out]
          }
          frame Enabled {
            # "#cruft removing I spectrum and Q spectrum\nat Nick's request. Using a disable structure for now,\nbecause we've reversed course on this multiple times already. Luke 1-8-2021"
          }
        }
        n53 = Bundle By Name(cluster=T1 {"Group_ref"=0, "TImeStamp_dset"=0, "PwrSpect_dset"=0, "ISpect_dset"=0, "QSpect_dset"=0} ("Complex"), "PwrSpect_dset"=w104, "ISpect_dset"=w103, "QSpect_dset"=w91) -> (w94:T1)
      }
    }
    frame True {
      n54 = for {
        tunnel: w611 -> [w635]
        shift-right: [w641] -> w609
        shift-left: w612 -> [w671]
        tunnel: w610 -> [w637] mode=indexing
        tunnel: [w644] -> w613 mode=indexing
        tunnel: w608 -> [w667]
        tunnel: w607 -> [w666]
        tunnel: w606 -> [w663]
        tunnel: w605 -> [w662]
        tunnel: w604 -> [w650]
        tunnel: w603 -> [w649]
        tunnel: w602 -> [w648]
        tunnel: [w642] -> w601 mode=indexing
        tunnel: w600 -> [w640]
        tunnel: w599 -> [w633]
        tunnel: w598 -> [w624]
        tunnel: w597 -> [w623]
        tunnel: w596 -> [w620]
        i -> [w614]
        # "Don't log peak location for \nCross channels. \nThey are duplicates of Co\nchannels."
        # "Only write Downshift with\nCo Channels."
        # "Only write DeltaPhase with \nCross Channels."
        # "Do these steps when we want to create a Dataset"
        # "Create Datasets\naka \"tables\" and\nsave refs to each.\nRepeat for each Tone"
        # "Set up Zoom arrays\n(each is 1D array of 1024 bins)\n100000 records planned\n(assuming about 84600\nrecords per day, at 1\nrecord per second)."
        # "set up Cal/Beac Datasets\n(each is a single cluster)\n100000 records planned\n(assuming about 84600\nrecords per day, at 1\nrecord per second)."
        # "open a Group\ni.e., Tone1"
        n55 = call <vilib>:"H5Gopen.vi"("create? (F)"=FALSE, "error in (no error)"=w671, "name"=w637, "ref in"=w635) -> ("error out"=w645:errorcluster, "group out"=w617:T2)  [unwired: 6 in]
        n56 = Bundle By Name(cluster=T3 {"Group_ref"=0, "Cal"={"TimeString_dset"=0, "TImeStamp_dset"=0, "SNR_dset"=0, "MaxValue_dset"=0, "PeakLoc_dset"=0, "df_dset"=0, "Phase_dset"=0, "DeltaPhase_dset"=0, "Downshift_dset"=0}, "Beac"={"TimeString_dset"=0, "TImeStamp_dset"=0, "SNR_dset"=0, "MaxValue_dset"=0, "PeakLoc_dset"=0, "df_dset"=0, "Phase_dset"=0, "DeltaPhase_dset"=0, "Downshift_dset"=0}, "CalZoom_dSet"=0, "BeacZoom_dSet"=0} ("Cluster"), "Group_ref"=w617) -> (w661:T3)
        n57 = call <vilib>:"H5Dopen.vi"("error in (no error)"=w645, "name"=w663, "loc in"=w617) -> ("error out"=w658:errorcluster, "dset out"=w660:T2)  [unwired: 7 in]
        n58 = case shown="0, 2" w614 {
          tunnel: w662 -> [_ w679]
          tunnel: [T2 0 ("dset out") w678] -> w659
          tunnel: w658 -> [w673 w677]
          tunnel: [w673 w676] -> w628
          tunnel: w617 -> [_ w675]
          frame Default {
          }
          frame 0, 2 {
            n59 = call <vilib>:"H5Dopen.vi"("error in (no error)"=w677, "name"=w679, "loc in"=w675) -> ("error out"=w676:errorcluster, "dset out"=w678:T2)  [unwired: 7 in]
          }
        }
        n60 = call "PushToErrorHandler.vi"("ErrorIn"=w628, "ErrorLocation"="LogReOpenCal") -> ("ErrorOut"=w615:errorcluster)  [unwired: 5 in]
        n61 = Bundle By Name(cluster=T4 {"TimeString_dset"=0, "TImeStamp_dset"=0, "SNR_dset"=0, "MaxValue_dset"=0, "PeakLoc_dset"=0, "df_dset"=0, "Phase_dset"=0, "DeltaPhase_dset"=0, "Downshift_dset"=0} ("Cal"), "MaxValue_dset"=w660, "PeakLoc_dset"=w659) -> (w665:T4)
        n62 = Bundle By Name(cluster=w661, "Cal"=w665) -> (w647:T3)
        n63 = call <vilib>:"H5Dopen.vi"("error in (no error)"=w615, "name"=w650, "loc in"=w617) -> ("error out"=w657:errorcluster, "dset out"=w653:T2)  [unwired: 7 in]
        n64 = call <vilib>:"H5Dopen.vi"("error in (no error)"=w657, "name"=w649, "loc in"=w617) -> ("error out"=w656:errorcluster, "dset out"=w654:T2)  [unwired: 7 in]
        n65 = case shown="Default" w614 {
          tunnel: w656 -> [w680 w686]
          tunnel: [T2 0 ("dset out") w685] -> w655
          tunnel: w648 -> [_ w684]
          tunnel: [w680 w683] -> w619
          tunnel: w617 -> [_ w682]
          frame Default {
          }
          frame 0, 2 {
            n66 = call <vilib>:"H5Dopen.vi"("error in (no error)"=w686, "name"=w684, "loc in"=w682) -> ("error out"=w683:errorcluster, "dset out"=w685:T2)  [unwired: 7 in]
          }
        }
        n67 = case shown="0, 2" w614 {
          tunnel: w620 -> [_ w693]
          tunnel: w619 -> [w687 w692]
          tunnel: [w687 w691] -> w618
          tunnel: w617 -> [_ w690]
          tunnel: [T2 0 ("dset out") w689] -> w616
          frame Default {
          }
          frame 0, 2 {
            n68 = call <vilib>:"H5Dopen.vi"("error in (no error)"=w692, "name"=w693, "loc in"=w690) -> ("error out"=w691:errorcluster, "dset out"=w689:T2)  [unwired: 7 in]
          }
        }
        n69 = call <vilib>:"H5Dopen.vi"("error in (no error)"=w618, "name"=w633, "loc in"=w617) -> ("error out"=w627:errorcluster, "dset out"=w632:T2)  [unwired: 7 in]
        n70 = call <vilib>:"H5Dopen.vi"("error in (no error)"=w627, "name"=w624, "loc in"=w617) -> ("error out"=w626:errorcluster, "dset out"=w622:T2)  [unwired: 7 in]
        n71 = case shown="1, 3" w614 {
          tunnel: w626 -> [w711 w716]
          tunnel: [w711 w715] -> w625
          tunnel: w623 -> [_ w714]
          tunnel: w617 -> [_ w713]
          tunnel: [T2 0 ("dset out") w712] -> w621
          frame Default {
          }
          frame 1, 3 {
            n72 = call <vilib>:"H5Dopen.vi"("error in (no error)"=w716, "name"=w714, "loc in"=w713) -> ("error out"=w715:errorcluster, "dset out"=w712:T2)  [unwired: 7 in]
          }
        }
        n73 = Bundle By Name(cluster=T4 {"TimeString_dset"=0, "TImeStamp_dset"=0, "SNR_dset"=0, "MaxValue_dset"=0, "PeakLoc_dset"=0, "df_dset"=0, "Phase_dset"=0, "DeltaPhase_dset"=0, "Downshift_dset"=0} ("Cal"), "TImeStamp_dset"=w653, "MaxValue_dset"=w654, "PeakLoc_dset"=w655, "Downshift_dset"=w616, "SNR_dset"=w632, "Phase_dset"=w622, "DeltaPhase_dset"=w621) -> (w651:T4)
        n74 = call "PushToErrorHandler.vi"("ErrorIn"=w625, "ErrorLocation"="LogReOpenBeac") -> ("ErrorOut"=w631:errorcluster)  [unwired: 5 in]
        n75 = Bundle By Name(cluster=w647, "Beac"=w651) -> (w644:T3)
        n76 = call <vilib>:"H5Gopen.vi"("create? (F)"=FALSE, "error in (no error)"=w631, "name"=w637, "ref in"=w635) -> ("error out"=w638:errorcluster, "group out"=w634:T2)  [unwired: 6 in]
        n77 = disable-structure shown="Enabled" {
          disable-tunnel: [w707 T2 0 ("dset out")] -> w670
          disable-tunnel: w667 -> [w706 _]
          disable-tunnel: [w705 w709] -> w646
          disable-tunnel: w638 -> [w704 w709]
          disable-tunnel: w634 -> [w703 _]
          frame Disabled {
            n78 = call <vilib>:"H5Dopen.vi"("error in (no error)"=w704, "name"=w706, "loc in"=w703) -> ("error out"=w705:errorcluster, "dset out"=w707:T2)  [unwired: 7 in]
          }
          frame Enabled {
          }
        }
        n79 = disable-structure shown="Enabled" {
          disable-tunnel: [w701 _] -> w669
          disable-tunnel: w666 -> [w700 _]
          disable-tunnel: w646 -> [w699 w702]
          disable-tunnel: [w697 w702] -> w641
          disable-tunnel: w640 -> [w696 _]
          disable-tunnel: [w695 _] -> w639
          disable-tunnel: w634 -> [w694 _]
          frame Disabled {
            n80 = call <vilib>:"H5Dopen.vi"("error in (no error)"=w699, "name"=w700, "loc in"=w694) -> ("error out"=w698:errorcluster, "dset out"=w701:T2)  [unwired: 7 in]
            n81 = call <vilib>:"H5Dopen.vi"("error in (no error)"=w698, "name"=w696, "loc in"=w694) -> ("error out"=w697:errorcluster, "dset out"=w695:T2)  [unwired: 7 in]
          }
          frame Enabled {
            # "#cruft removing I spectrum and Q spectrum\nat Nick's request. Using a disable structure for now,\nbecause we've reversed course on this multiple times already. Luke 1-8-2021"
          }
        }
        n82 = Bundle By Name(cluster=T1 {"Group_ref"=0, "TImeStamp_dset"=0, "PwrSpect_dset"=0, "ISpect_dset"=0, "QSpect_dset"=0} ("Complex"), "Group_ref"=w634, "PwrSpect_dset"=w670, "ISpect_dset"=w669, "QSpect_dset"=w639) -> (w642:T1)
      }
    }
  }
  "ToneRefs" <- w22
  "ComplexRefs" <- w9
  n83 = call "PushToErrorHandler.vi"("ErrorIn"=w7, "ErrorLocation"="Log_InitTone") -> ("ErrorOut"=→"error out":errorcluster)  [unwired: 5 in]
  "HDF5 file ref" <- "HDF5 file ref"
